vi "SimpleGyroGlobal.vi"() -> ()   [LabVIEW 2014]
panel:
  in  "Gyro Reset":bool
  in  "Gyro Angle":dbl
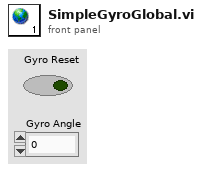
[diagram p1: front panel]
diagram:
